vi "GCSArray_valid_file.vi"(0 "GCS Array Filepath":path, 5 "error in (no error)":errorcluster, 6 "Block index":i32 min=0 max=0) -> (14 "Is valid?":bool, 19 "error out":errorcluster)   [LabVIEW 2026]
doc: "Load specified GCSArray from file into 2D double array."
uses:
  GCSArray_regex_selector.ctl
  GCSArray_regex_range.ctl
panel:
  out "Failed condition":string
  in  "Throw on Error?":bool
  # "Runs validity checks on GCSArray file to verify\nif it contains a valid GCS Array Data Format Description\n(Release 1.2.1, Date: 2010-09-27, PI document code SM146E).\nIn case the validation fails, the text field 'Failed condition'\ncontains a human readable error description."
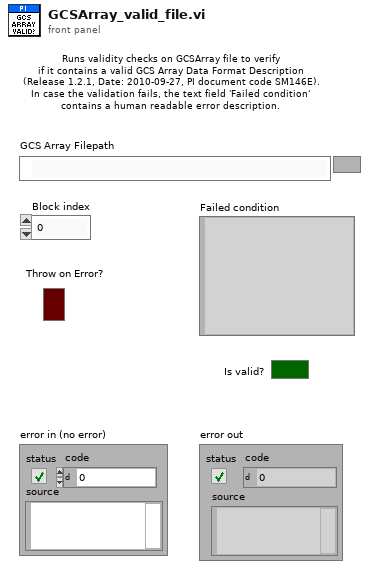
[diagram p1: front panel]
types:
  T1 = typedef "GCSArray_regex_range.ctl" = cluster{"Begin":i32, "End":i32}
  T2 = typedef "GCSArray_regex_selector.ctl" = enum16{"GCS_ARRAY Block Full", "GCS_ARRAY Block ID", "GCS_ARRAY Block Header", "GCS_ARRAY Block Data", "GCS_ARRAY Identifier", "GCS_ARRAY Remark", "GCS_ARRAY Version", "GCS_ARRAY Dimension", "GCS_ARRAY Type", "GCS_ARRAY Separator", "GCS_ARRAY NData", "GCS_ARRAY NData%", "GCS_ARRAY NData% Keyword", "GCS_ARRAY Name%", "GCS_ARRAY Name% Keyword", "GCS_ARRAY Start%", "GCS_ARRAY Start% Keyword", "GCS_ARRAY End%", "GCS_ARRAY End% Keyword", "GCS_ARRAY Delta%", "GCS_ARRAY Delta% Keword", "GCS_ARRAY Sample Time", "GCS_ARRAY Unit of transmitted value%", "GCS_ARRAY Trans_Unit% Keyword", "GCS_ARRAY Trans_Unit% = RAW Keyword", "GCS_ARRAY Unit of displayed value%", "GCS_ARRAY Disp_Unit% Keyword", "GCS_ARRAY Nominator%", "GCS_ARRAY Ratio_Nom% Keyword", "GCS_ARRAY Denominator%", "GCS_ARRAY Ratio_Denom% Keyword", "GCS_ARRAY End of Header", "GCS_ARRAY Empty line of Header"}
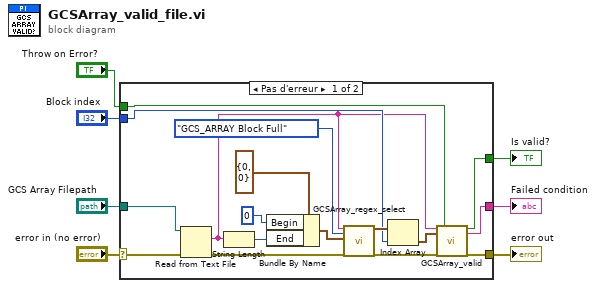
[diagram p0: block diagram]
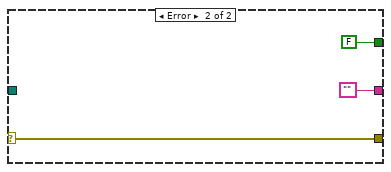
[diagram p2: hidden frame]
diagram:
  n1 = case shown="Pas d'erreur" "error in (no error)" {
    selector: "error in (no error)" -> [w23 w27]
    tunnel: [w12 w27] -> w6
    tunnel: "Block index" -> [w16 _]
    tunnel: "GCS Array Filepath" -> [w24 _]
    tunnel: "Throw on Error?" -> [w13 _]
    tunnel: [w11 ""] -> w2
    tunnel: [w10 FALSE ("Is valid?")] -> w1
    frame No Error {
      n2 = Read from Text File(file (use dialog)=w24, error in=w23) -> (text=w9:string, error out=w19:errorcluster)  [unwired: 4 out]
      n3 = String Length(string=w9) -> (length=w20:i32)
      n4 = Bundle By Name(cluster=T1 {"Begin"=0, "End"=0} ("Selection"), "Begin"=0, "End"=w20) -> (w15:T1)
      n5 = call "GCSArray_regex_select.vi"("GCSArray input string"=w9, "Selector"=GCSArray_regex_selector."GCS_ARRAY Block Full", "Range"=w15, "error in (no error)"=w19) -> ("Matches"=w17:T1[], "error out"=w18:errorcluster)  [unwired: 14 out]
      n6 = Index Array(array=w17, index=w16) -> (element=w8:T1)
      n7 = call "GCSArray_valid.vi"("GCSArray input string"=w9, "Selection"=w8, "error in (no error)"=w18, "Throw on Error?"=w13) -> ("Is valid?"=w10:bool, "Failed condition"=w11:string, "error out"=w12:errorcluster)  [unwired: 13 in]
    }
    frame Error {
    }
  }
  "error out" <- w6
  "Is valid?" <- w1
  "Failed condition" <- w2
